vi "Commit Move.vi"(8 "error in (no error)":errorcluster, 11 "Game Engine in":refnum<class "Game Engine.lvclass">) -> (0 "error out":errorcluster, 3 "Game Engine out":refnum<class "Game Engine.lvclass">)   [LabVIEW 2017, in "Game Engine.lvlib" / "Game Engine.lvclass"]
uses:
  Game Engine.lvclass
  Game Engine.lvclass/Game Engine.ctl
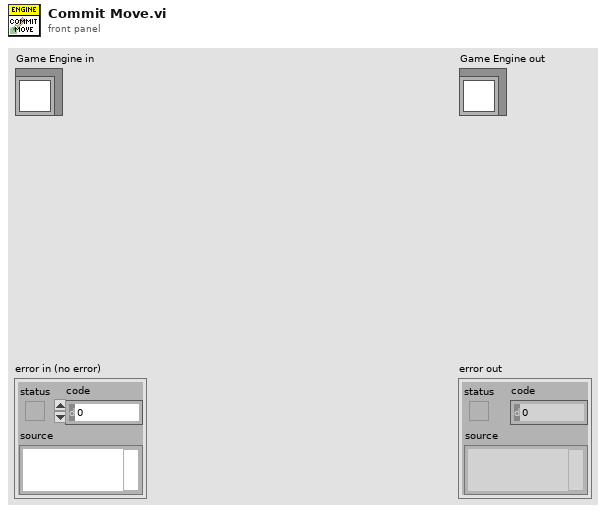
[diagram p1: front panel]
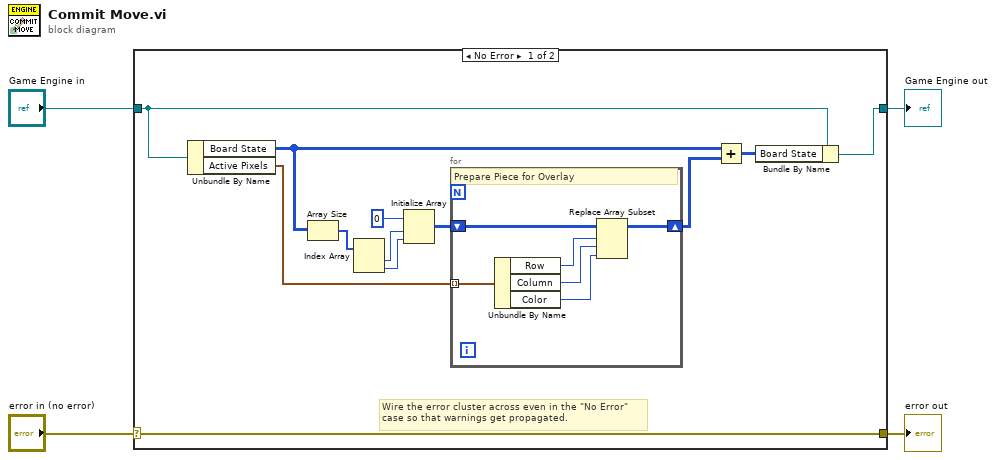
[diagram p0: block diagram]
diagram:
  n1 = case shown="No Error" "error in (no error)" {
    selector: "error in (no error)" -> [w16 w24]
    tunnel: [w16 w24] -> w3
    tunnel: [w5 w23] -> w1
    tunnel: "Game Engine in" -> [w7 w23]
    frame No Error {
      # "Wire the error cluster across even in the \"No Error\"\ncase so that warnings get propagated."
      n2 = Unbundle By Name(w7) -> ("Board State"=w9:u32[][], "Active Pixels"=w13:cluster{"Column":u8, "Row":u8, "Color":u32}[])
      n3 = Array Size(array=w9) -> (size(s)=w12:i32[])
      n4 = Index Array(array=w12) -> (element #1=w11:i32, element #2=w10:i32)  [unwired: 2 in]
      n5 = Initialize Array(u32 0, w11, w10) -> (w14:u32[][])
      n6 = for {
        tunnel: w13 -> [w22] mode=indexing
        shift-right: [w17] -> w8
        shift-left: w14 -> [w21]
        # "Prepare Piece for Overlay"
        n7 = Unbundle By Name(w22) -> ("Row"=w20:u8, "Column"=w19:u8, "Color"=w18:u32)
        n8 = Replace Array Subset(array=w21, new element=w18, index (row)=w20, index (col)=w19) -> (w17:u32[][])
      }
      n9 = Add(x=w9, y=w8) -> (x+y=w6:u32[][])
      n10 = Bundle By Name(cluster=w7, "Board State"=w6) -> (w5:refnum<class "Game Engine.lvclass">)
    }
    frame Error {
    }
  }
  "error out" <- w3
  "Game Engine out" <- w1
